vi "Write to DB.vi"(8 "error in (no error)":errorcluster, 11 "Database Entry in":refnum<class "Database Entry.lvclass">) -> (0 "error out":errorcluster, 3 "Database Entry out":refnum<class "Database Entry.lvclass">)   [LabVIEW 2021, in "Database Entry.lvclass"]
uses:
  Database Entry.lvclass
  Database Entry.lvclass/Database Entry.ctl
  <vilib>/Utility/file.llb/Read Delimited Spreadsheet (string).vi
  Stack/Stack.lvclass
panel:
  out "Data cluster":T1={"type"="proto", " geometry"="full", "resolution"="LD", "baselayer"="BA_123", "toplayer"="SI_789", "bl_pos"="1", "tl_pos"="1", "put_pos"="1", "region"="1", "asstray"="1", "comptray"="1", "put"="1", "date"="2024-04-02", "timestart"="1:12:12.442", "timeend"="1:23:45.244", "operator"="cmuperson", "tape"="some", "glue"="some", "stack name"="some"}
  out "error out py":errorcluster
  in  "function name":string="assembly_data"
  out "String Out":string="Upload Success"
  in  "Python version":string="3.7.0"
  in  "error in (no error) py":errorcluster
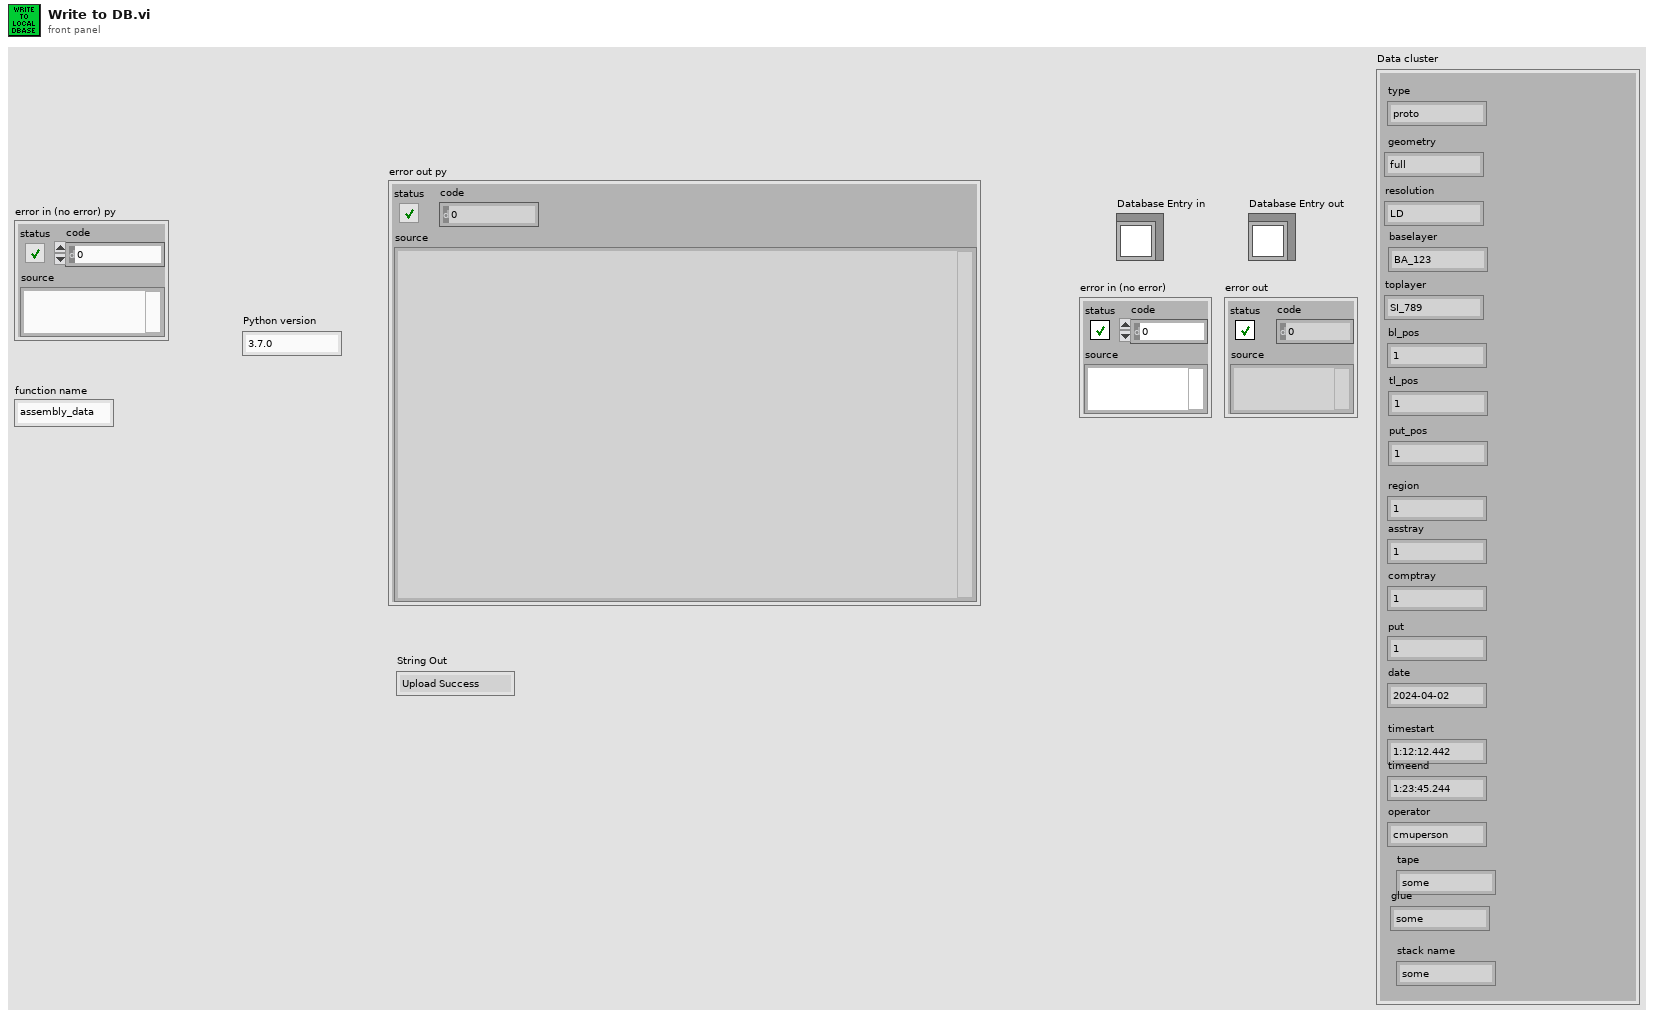
[diagram p1: front panel]
types:
  T1 = cluster{"type":string, " geometry":string, "resolution":string, "baselayer":string, "toplayer":string, "bl_pos":string, "tl_pos":string, "put_pos":string, "region":string, "asstray":string, "comptray":string, "put":string, "date":string, "timestart":string, "timeend":string, "operator":string, "tape":string, "glue":string, "stack name":string}
  T2 = typedef "File Paths.ctl" = cluster{"Glue Pattern Folder":path, "Carrier Tray Folder":path, "Pick Up Tool Fixture Folder":path, "Components Folder":path, "Bellows Tool Offset.txt":path, "Pick Up Tool Offset.txt":path, "Dispense Tip Offset.txt":path, "Log Files":path, "Gantry Assembly Map.txt":path, "Syringe and offset map.txt":path, "Python DB Conn":path}
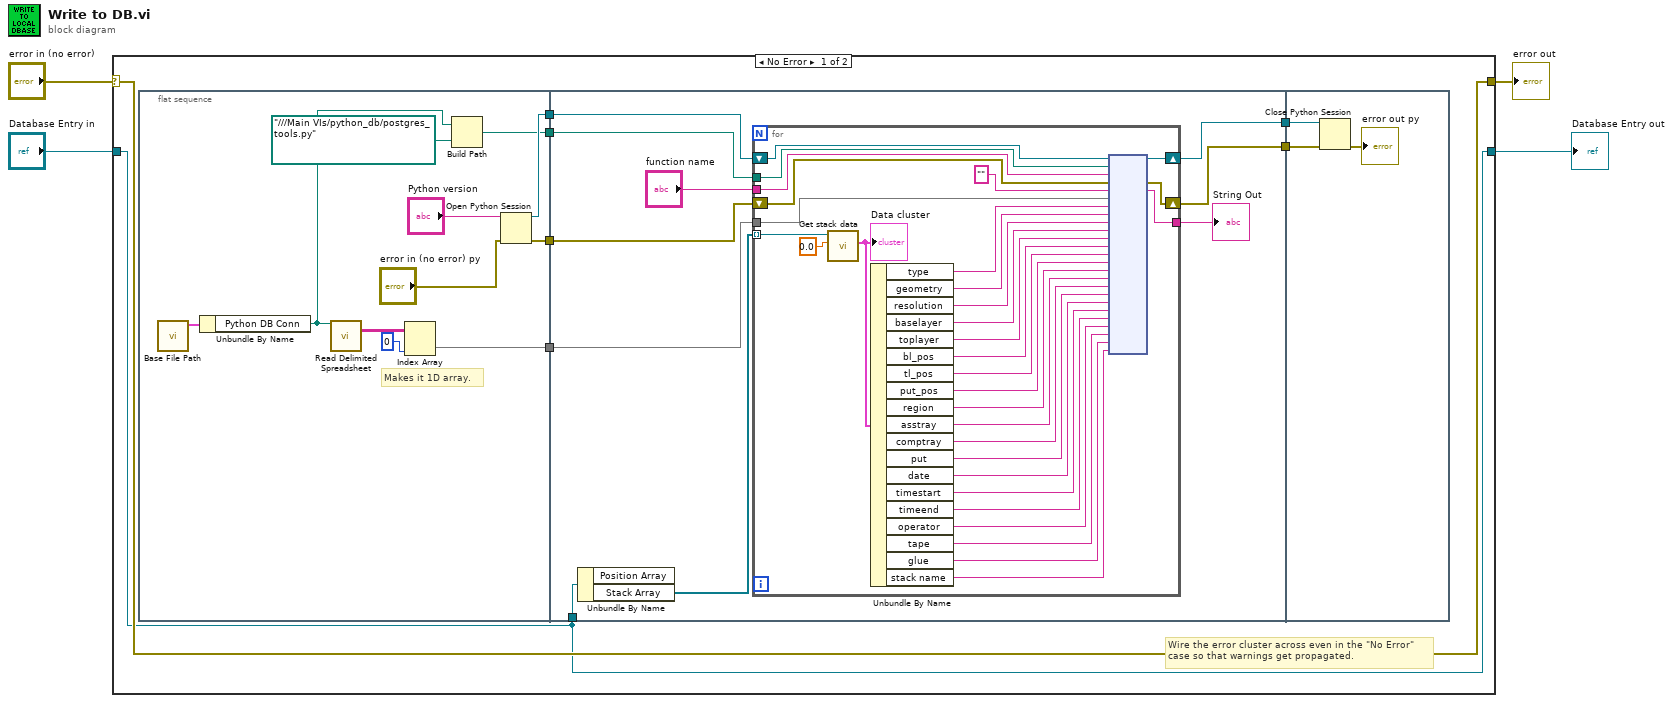
[diagram p0: block diagram]
diagram:
  n1 = case shown="No Error" "error in (no error)" {
    selector: "error in (no error)" -> [w12 w69]
    tunnel: [w12 w69] -> w3
    tunnel: [w5 w68] -> w1
    tunnel: "Database Entry in" -> [w5 w68]
    frame No Error {
      # "Wire the error cluster across even in the \"No Error\"\ncase so that warnings get propagated."
      n2 = flat-sequence {
        tunnel: [w22] -> w11
        tunnel: [w23] -> w10
        tunnel: [w18] -> w9
        tunnel: [w14] -> w8
        tunnel: [w32] -> w7
        tunnel: [w31] -> w6
        tunnel: w11 -> [w33]
        tunnel: w10 -> [w30]
        tunnel: w9 -> [w29]
        tunnel: w8 -> [w28]
        tunnel: w5 -> [w27]
        tunnel: w7 -> [w66]
        tunnel: w6 -> [w67]
        frame #0 {
          # "Makes it 1D array."
          n3 = call "Base File Path.vi"() -> ("Paths Out"=w19:T2)  [unwired: 11 in]
          n4 = Unbundle By Name(w19) -> ("Python DB Conn"=w17:path)
          n5 = call-poly <vilib>:"Read Delimited Spreadsheet.vi"("file path (dialog if empty)"=w17) -> ("all rows"=w16:string[][])  [unwired: 9 in, 5 out]
          n6 = Index Array(array=w16, index (col)=0 ("disabled index (col)")) -> (element=w14:string[])  [unwired: 1 in]
          n7 = Build Path(base path=w17, name or relative path=path "../../../Main VIs/python_db/postgres_tools.py" ("module path")) -> (appended path=w18:path)
          n8 = Open Python Session(python version="Python version", 3:"error in (no error) py") -> (session out=w23:refnum<k35>, error out=w22:errorcluster)  [unwired: 1 in]
        }
        frame #1 {
          n9 = Unbundle By Name(w27) -> ("Stack Array"=w24:refnum<class "Stack.lvclass">[])  [unwired: 1 out]
          n10 = for {
            tunnel: w29 -> [w60]
            shift-right: [w63] -> w32
            shift-left: w33 -> [w64]
            shift-right: [w62] -> w31
            shift-left: w30 -> [w61]
            tunnel: "function name" -> [w59]
            tunnel: [w57] -> w25
            tunnel: w24 -> [w56] mode=indexing
            tunnel: w28 -> [w55]
            n11 = call "Get stack data.vi"("Last Index for Type"=0.0, "Stack in"=w56) -> ("Data cluster"=w53:T1)  [unwired: 7 in, 2 out]
            "Data cluster" <- w53
            n12 = Unbundle By Name(w53) -> ("type"=w52:string, "geometry"=w51:string, "resolution"=w50:string, "baselayer"=w49:string, "toplayer"=w48:string, "bl_pos"=w47:string, "tl_pos"=w46:string, "put_pos"=w45:string, "region"=w44:string, "asstray"=w43:string, "comptray"=w42:string, "put"=w41:string, "date"=w40:string, "timestart"=w39:string, "timeend"=w38:string, "operator"=w37:string, "tape"=w36:string, "glue"=w35:string, "stack name"=w34:string)
            n13 = node(w61, w60, w59, w64, "", w55, w52, w51, w50, w49, w48, w47, w46, w45, w44, w43, w42, w41, w40, w39, w38, w37, w36, w35, w34) -> (w62:refnum<k35>, w63:errorcluster, w57:string)  [unwired: 20 in, 2 out]
          }
          "String Out" <- w25
        }
        frame #2 {
          n14 = Close Python Session(session in=w67, error in=w66) -> (11:→"error out py":errorcluster)
        }
      }
    }
    frame Error {
    }
  }
  "error out" <- w3
  "Database Entry out" <- w1
